vi "Get Limit Value String.vi"(8 "error in (no error)":errorcluster, 9 "Limit":enum16{"LIMIT1", "LIMIT2"}(ring), 10 "Step Output in":T1, 11 "Execution in":refnum<data-value>) -> (0 "error out":errorcluster, 2 "Limit Value":string, 3 "Execution out":refnum<data-value>)   [LabVIEW 2015, in "Execution.lvclass"]
uses:
  Execution.lvclass
  Step/STEP_OUTPUT.ctl
  Step/OUTPUT_DATA_TYPE.ctl
  OutputUI/OUTPUT_CHECK_TYPE.ctl
  Step/OUTPUT_VALUE_TYPE.ctl
  Step.lvclass
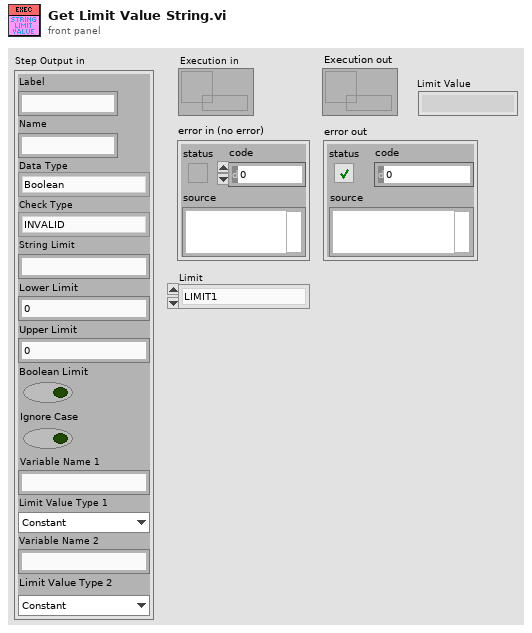
[diagram p1: front panel]
types:
  T1 = typedef "Step.lvclass/STEP_OUTPUT.ctl" = cluster{"Label":string, "Name":string, "Data Type":T2, "Check Type":T3, "String Limit":string, "Lower Limit":dbl, "Upper Limit":dbl, "Boolean Limit":bool, "Ignore Case":bool, "Variable Name 1":string, "Limit Value Type 1":T4, "Variable Name 2":string, "Limit Value Type 2":T4}
  T2 = typedef "Step.lvclass/OUTPUT_DATA_TYPE.ctl" = enum16{"Boolean", "String", "Numeric", "Other"}
  T3 = typedef "Step.lvclass/OUTPUT_CHECK_TYPE.ctl" = enum16{"INVALID", "DO_NOT_CHECK", "RECORD", "VARIABLE", "EQUAL", "NOT_EQUAL", "STR_CONTAINS", "STR_START_WITH", "STR_END_WITH", "STR_REGEX_MATCH", "NUM_GT", "NUM_LT", "NUM_GE", "NUM_LE", "NUM_RANGE", "NUM_RANGE_BDY"}
  T4 = typedef "Step.lvclass/OUTPUT_VALUE_TYPE.ctl" = enum16{"Constant", "Variable"}
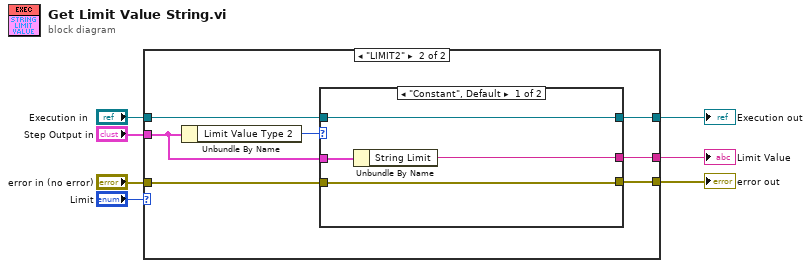
[diagram p0: block diagram]
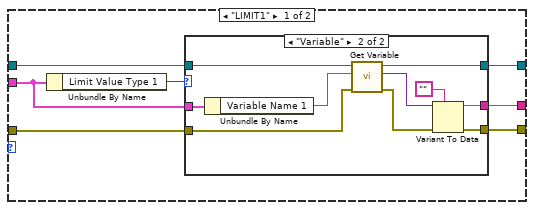
[diagram p2: hidden frame]
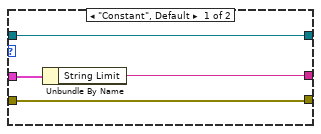
[diagram p3: hidden frame]
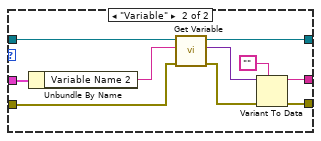
[diagram p4: hidden frame]
diagram:
  n1 = case shown="\"LIMIT2\"" "Limit" {
    tunnel: "Step Output in" -> [w14 w35]
    tunnel: "Execution in" -> [w12 w33]
    tunnel: [w11 w32] -> w5
    tunnel: [w10 w31] -> w4
    tunnel: [w9 w30] -> w3
    tunnel: "error in (no error)" -> [w8 w29]
    frame "LIMIT1" {
      n2 = Unbundle By Name(w14) -> ("Limit Value Type 1"=w13:T4)
      n3 = case shown="\"Variable\"" w13 {
        tunnel: w12 -> [w17 w28]
        tunnel: [w17 w27] -> w11
        tunnel: w14 -> [w18 w21]
        tunnel: [w16 w23] -> w10
        tunnel: [w15 w22] -> w9
        tunnel: w8 -> [w15 w19]
        frame "Constant", Default {
          n4 = Unbundle By Name(w18) -> ("String Limit"=w16:string)
        }
        frame "Variable" {
          n5 = Unbundle By Name(w21) -> ("Variable Name 1"=w20:string)
          n6 = call "Get Variable.vi"("error in (no error)"=w19, "Name"=w20, "Execution in"=w28) -> ("error out"=w26:errorcluster, "Value"=w25:variant, "Execution out"=w27:refnum<data-value>)  [unwired: 6 in]
          n7 = Variant To Data(error in=w26, type="", Variant=w25) -> (data=w23:string, error out=w22:errorcluster)
        }
      }
    }
    frame "LIMIT2" {
      n8 = Unbundle By Name(w35) -> ("Limit Value Type 2"=w34:T4)
      n9 = case shown="\"Constant\", Default" w34 {
        tunnel: w33 -> [w38 w49]
        tunnel: [w38 w48] -> w32
        tunnel: w35 -> [w39 w42]
        tunnel: [w37 w44] -> w31
        tunnel: [w36 w43] -> w30
        tunnel: w29 -> [w36 w40]
        frame "Constant", Default {
          n10 = Unbundle By Name(w39) -> ("String Limit"=w37:string)
        }
        frame "Variable" {
          n11 = Unbundle By Name(w42) -> ("Variable Name 2"=w41:string)
          n12 = call "Get Variable.vi"("error in (no error)"=w40, "Name"=w41, "Execution in"=w49) -> ("error out"=w47:errorcluster, "Value"=w46:variant, "Execution out"=w48:refnum<data-value>)  [unwired: 6 in]
          n13 = Variant To Data(error in=w47, type="", Variant=w46) -> (data=w44:string, error out=w43:errorcluster)
        }
      }
    }
  }
  "Execution out" <- w5
  "Limit Value" <- w4
  "error out" <- w3
